vi "Save1DWaveformToFile.vi"(6 "header? (write header:T)":bool=TRUE, 7 "delimiter (Tab)":string="\t", 8 "error in (no error)":errorcluster, 9 "multiple time columns? (single:F)":bool, 10 "waveforms":waveform(dbl)[](array[waveform]), 11 "refnum":refnum<file>) -> (0 "error out":errorcluster, 3 "dup refnum":refnum<file>)   [LabVIEW 2022 SP3]
uses:
  <vilib>/Waveform/WDTOps.llb/WDT Get Waveform Time Array DBL.vi
panel:
  out "spreadsheet string":string
  out "Array":string[](array[string])
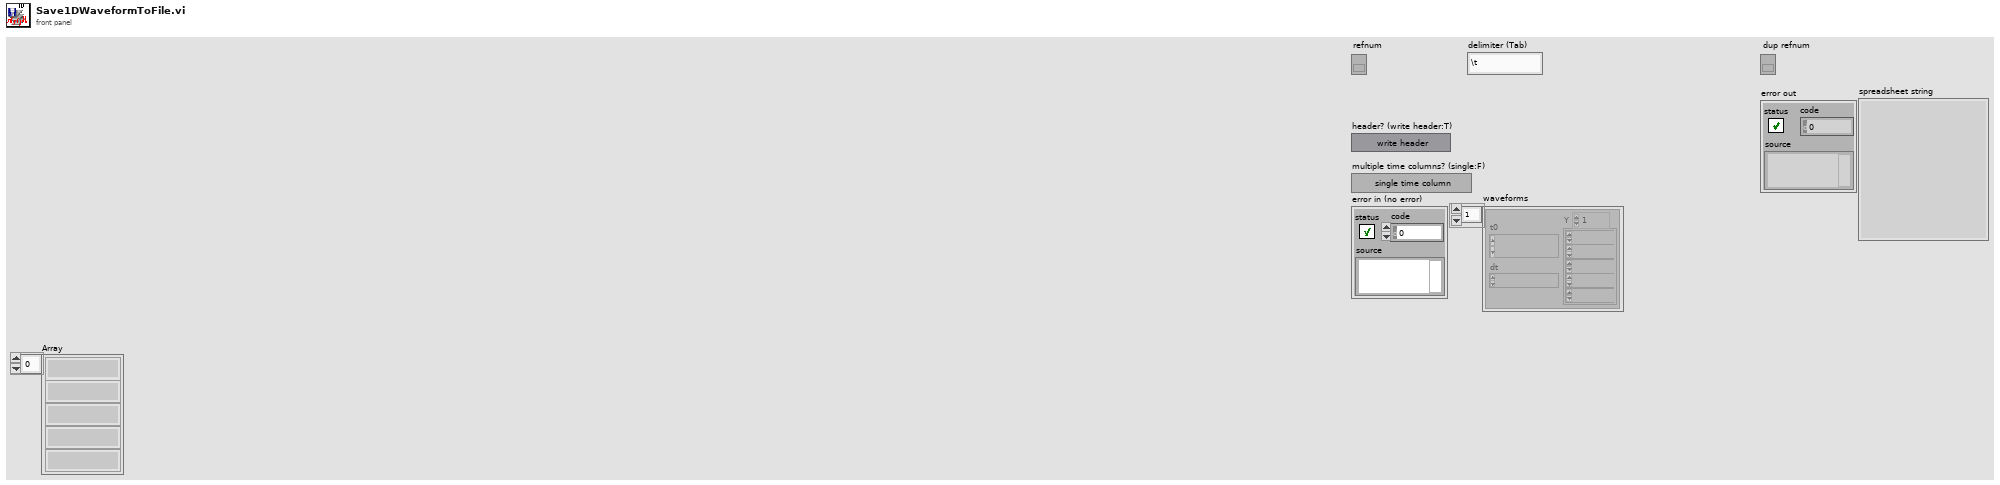
[diagram p1: front panel]
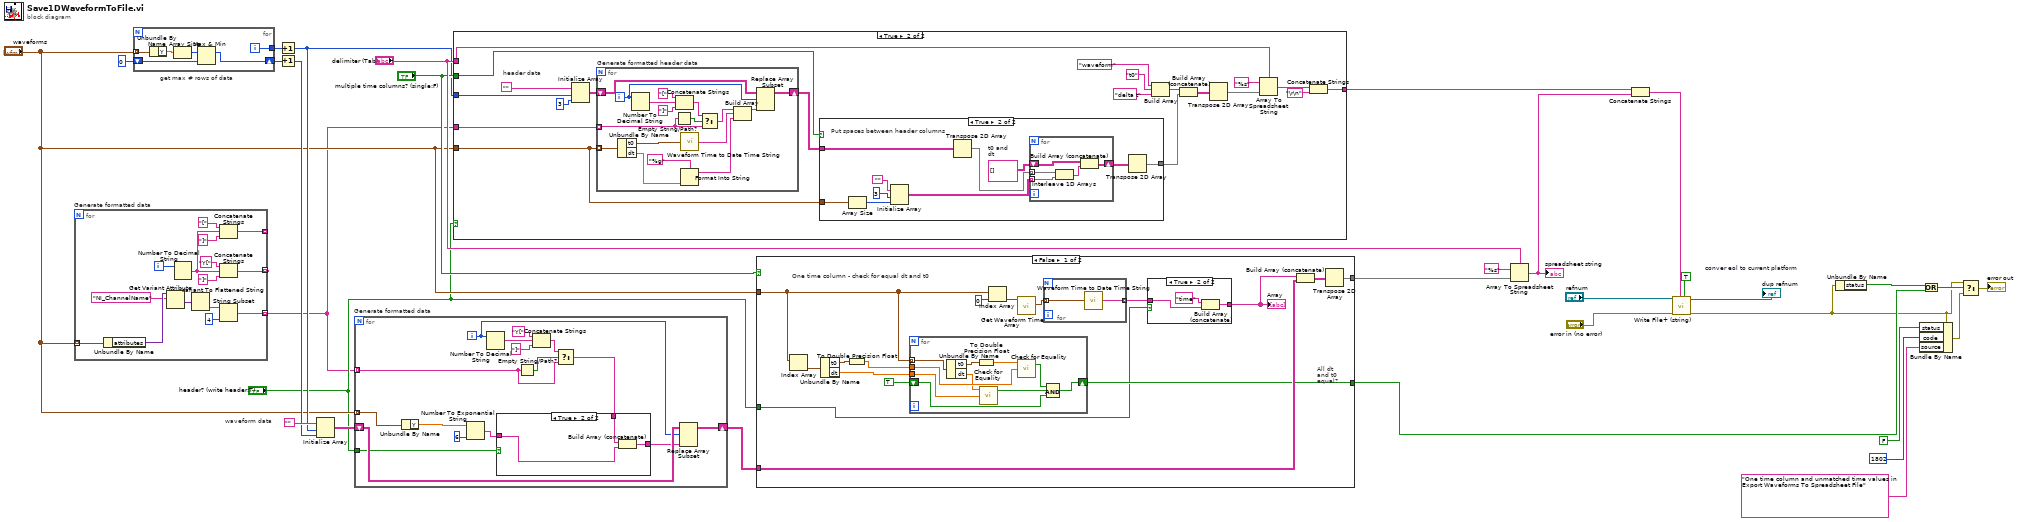
[diagram p0: block diagram]
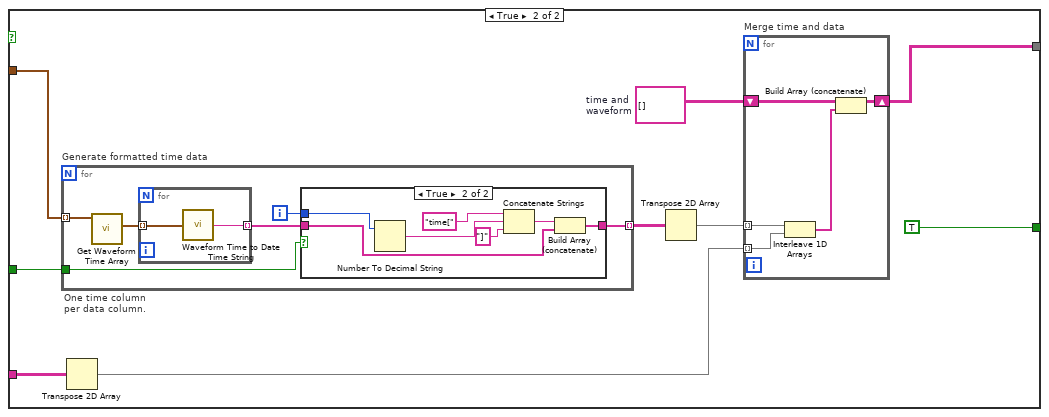
[diagram p3: hidden frame]
diagram:
  w30 = TRUE  # conver eol to current platform
  # "waveform data"
  # "get max # rows of data"
  n1 = for "Generate formatted data" {
    tunnel: "waveforms" -> [w46] mode=indexing
    tunnel: [w37] -> _ mode=indexing
    tunnel: [w36] -> w4 mode=indexing
    tunnel: [w32] -> _ mode=indexing
    i -> [w38]
    n2 = Unbundle By Name(w46) -> ("attributes"=w43:variant)
    n3 = Get Variant Attribute(Variant=w43, name="NI_ChannelName") -> (value=w41:variant)  [unwired: 2 in, 3 out]
    n4 = Number To Decimal String(number=w38) -> (decimal integer string=w33:string)  [unwired: 1 in]
    n5 = Variant To Flattened String(Variant=w41) -> (data string=w44:string)  [unwired: 1 out]
    n6 = String Subset(string=w44, offset (0)=4) -> (substring=w36:string)  [unwired: 1 in]
    n7 = Concatenate Strings("[", w33, "]") -> (w32:string)
    n8 = Concatenate Strings("Y[", w33, "]") -> (w37:string)
  }
  n9 = for {
    tunnel: "waveforms" -> [w52] mode=indexing
    shift-right: [w48] -> w11
    shift-left: 0 -> [w49]
    tunnel: [w47] -> w9
    i -> [w47]
    n10 = Unbundle By Name(w52) -> ("Y"=w51:dbl[])
    n11 = Array Size(array=w51) -> (size(s)=w50:i32)
    n12 = Max & Min(x=w50, y=w49) -> (max(x,y)=w48:i32)  [unwired: 1 out]
  }
  n13 = Increment(x=w9) -> (x+1=w8:i32)
  n14 = Increment(x=w11) -> (x+1=w7:i32)
  n15 = Initialize Array("", w8, w7) -> (w10:string[][])
  n16 = for "Generate formatted data" {
    tunnel: "waveforms" -> [w66] mode=indexing
    tunnel: "header? (write header:T)" -> [w63]
    shift-right: [w64] -> w24
    shift-left: w10 -> [w65]
    tunnel: w4 -> [w53] mode=indexing
    i -> [w55]
    n17 = Unbundle By Name(w66) -> ("Y"=w68:dbl[])
    n18 = Number To Exponential String(number=w68, precision (6)=i16 6) -> (E-format string=w62:string[])  [unwired: 2 in]
    n19 = Number To Decimal String(number=w55) -> (decimal integer string=w60:string)  [unwired: 1 in]
    n20 = Empty String/Path?(string/path=w53) -> (empty?=w57:bool)
    n21 = Concatenate Strings("Y[", w60, "]") -> (w54:string)
    n22 = Select(t=w54, s=w57, f=w53) -> (s? t:f=w56:string)
    n23 = case shown="True" w63 {
      tunnel: w62 -> [w69 w72]
      tunnel: [w69 w71] -> w61
      tunnel: w56 -> [_ w70]
      frame False {
      }
      frame True {
        n24 = Build Array (concatenate)(w70, w72) -> (w71:string[])
      }
    }
    n25 = Replace Array Subset(array=w65, new element=w61, index (row)=w55) -> (w64:string[][])  [unwired: 1 in]
  }
  n26 = case shown="True" "header? (write header:T)" {
    tunnel: "delimiter (Tab)" -> [_ w90]
    tunnel: "waveforms" -> [_ w84]
    tunnel: [_ w85] -> w25
    tunnel: "multiple time columns? (single:F)" -> [_ w82]
    tunnel: w8 -> [_ w75]
    tunnel: w4 -> [_ w73]
    frame False {
    }
    frame True {
      # "header data"
      n27 = Initialize Array("", w75, 3 ("dimension size")) -> (w74:string[][])
      n28 = for "Generate formatted header data" {
        tunnel: w84 -> [w119] mode=indexing
        shift-right: [w114] -> w80
        shift-left: w74 -> [w115]
        tunnel: w73 -> [w109] mode=indexing
        i -> [w113]
        n29 = Unbundle By Name(w119) -> ("t0"=w117:timestamp, "dt"=w123:dbl)
        n30 = Number To Decimal String(number=w113) -> (decimal integer string=w122:string)  [unwired: 1 in]
        n31 = Concatenate Strings("[", w122, "]") -> (w112:string)
        n32 = Empty String/Path?(string/path=w109) -> (empty?=w110:bool)
        n33 = call <vilib>:"Waveform Time to Date Time String.vi"("t0"=w117) -> ("String"=w124:string)
        n34 = Format Into String(format string="%g" ("Format String"), w123) -> (resulting string=w125:string)  [unwired: 2 in, 1 out]
        n35 = Select(t=w112, s=w110, f=w109) -> (s? t:f=w111:string)
        n36 = Build Array(w111, w124, w125) -> (w116:string[])
        n37 = Replace Array Subset(array=w115, new element=w116, index (row)=w113) -> (w114:string[][])  [unwired: 1 in]
      }
      n38 = case shown="True" w82 {
        tunnel: w84 -> [_ w103]
        tunnel: [w93 w98] -> w81
        tunnel: w80 -> [w93 w97]
        frame False {
          # "Leave the header data alone"
        }
        frame True {
          w101 = string[][] []  # t0 and dt
          # "Put spaces between header columns"
          n39 = Array Size(array=w103) -> (size(s)=w94:i32)
          n40 = Initialize Array("", 3 ("Dimension Size"), w94) -> (w100:string[][])
          n41 = Transpose 2D Array(2D array=w97) -> (transposed array=w96:string[][])
          n42 = for {
            shift-right: [w105] -> w99
            shift-left: w101 -> [w106]
            tunnel: w100 -> [w108] mode=indexing
            tunnel: w96 -> [w104] mode=indexing
            n43 = Interleave 1D Arrays(w104, w108) -> (w107:string[])
            n44 = Build Array (concatenate)(w106, w107) -> (w105:string[][])
          }
          n45 = Transpose 2D Array(2D array=w99) -> (transposed array=w98:string[][])
        }
      }
      n46 = Build Array("waveform", "t0", "delta t") -> (w83:string[])
      n47 = Build Array (concatenate)(w83, w81) -> (w78:string[][])
      n48 = Transpose 2D Array(2D array=w78) -> (transposed array=w79:string[][])
      n49 = Array To Spreadsheet String(delimiter (Tab)=w90, array=w79, 3:"%s" ("format string")) -> (spreadsheet string=w87:string)
      n50 = Concatenate Strings(w87, "\r\n") -> (w85:string)
    }
  }
  n51 = case shown="False" "multiple time columns? (single:F)" {
    tunnel: "waveforms" -> [w130 w166]
    tunnel: w24 -> [w137 w164]
    tunnel: [w135 w160] -> w23
    tunnel: [w129 TRUE] -> w14
    tunnel: "header? (write header:T)" -> [w126 w158]
    frame False {
      # "One time column - check for equal dt and t0"
      # "All dt\nand t0\nequal?"
      n52 = Index Array(array=w130) -> (element=w134:waveform(dbl))  [unwired: 1 in]
      n53 = Unbundle By Name(w134) -> ("t0"=w128:timestamp, "dt"=w131:dbl)
      n54 = To Double Precision Float(number=w128) -> (double precision float=w132:dbl)
      n55 = for {
        tunnel: w130 -> [w155] mode=indexing
        shift-right: [w150] -> w129
        shift-left: TRUE -> [w149]
        tunnel: w132 -> [w153]
        tunnel: w131 -> [w151]
        n56 = Unbundle By Name(w155) -> ("t0"=w146:timestamp, "dt"=w152:dbl)
        n57 = To Double Precision Float(number=w146) -> (double precision float=w154:dbl)
        n58 = call <vilib>:"Check for Equality.vi"("n2"=w151, "n1"=w152) -> ("equal?"=w148:bool)  [unwired: 1 in, 1 out]
        n59 = call <vilib>:"Check for Equality.vi"("n2"=w153, "n1"=w154) -> ("equal?"=w147:bool)  [unwired: 1 in, 1 out]
        n60 = Compound Arithmetic op=AND(w147, w148, w149) -> (w150:bool)
      }
      n61 = Index Array(array=w130, index=0 ("Index")) -> (element=w139:waveform(dbl))
      n62 = call-poly <vilib>:"Get Waveform Time Array.vi"("waveform in"=w139) -> ("X array"=w141:timestamp[])  [unwired: 9 in, 1 out]
      n63 = for {
        tunnel: w141 -> [w156] mode=indexing
        tunnel: [w157] -> w138 mode=indexing
        n64 = call <vilib>:"Waveform Time to Date Time String.vi"("t0"=w156) -> ("String"=w157:string)
      }
      n65 = case shown="True" w126 {
        tunnel: w138 -> [w142 w145]
        tunnel: [w142 w144] -> w127
        frame False {
        }
        frame True {
          n66 = Build Array (concatenate)("time", w145) -> (w144:string[])
        }
      }
      "Array" <- w127
      n67 = Build Array (concatenate)(w127, w137) -> (w136:string[][])
      n68 = Transpose 2D Array(2D array=w136) -> (transposed array=w135:string[][])
    }
    frame True {
      w161 = string[][] []  # time and waveform
      # "One time column\nper data column."
      n69 = for "Generate formatted time data" {
        tunnel: [w172] -> w165 mode=indexing
        tunnel: w166 -> [w176] mode=indexing
        tunnel: w158 -> [w174]
        i -> [w175]
        n70 = call-poly <vilib>:"Get Waveform Time Array.vi"("waveform in"=w176) -> ("X array"=w177:timestamp[])  [unwired: 9 in, 1 out]
        n71 = for {
          tunnel: w177 -> [w186] mode=indexing
          tunnel: [w187] -> w173 mode=indexing
          n72 = call <vilib>:"Waveform Time to Date Time String.vi"("t0"=w186) -> ("String"=w187:string)
        }
        n73 = case shown="True" w174 {
          tunnel: w175 -> [_ w182]
          tunnel: w173 -> [w178 w180]
          tunnel: [w178 w179] -> w172
          frame False {
          }
          frame True {
            n74 = Number To Decimal String(number=w182) -> (decimal integer string=w185:string)  [unwired: 1 in]
            n75 = Concatenate Strings("time[", w185, "]") -> (w181:string)
            n76 = Build Array (concatenate)(w181, w180) -> (w179:string[])
          }
        }
      }
      n77 = Transpose 2D Array(2D array=w164) -> (transposed array=w163:string[][])
      n78 = Transpose 2D Array(2D array=w165) -> (transposed array=w162:string[][])
      n79 = for "Merge time and data" {
        tunnel: w163 -> [w170] mode=indexing
        tunnel: w162 -> [w169] mode=indexing
        shift-right: [w168] -> w160
        shift-left: w161 -> [w171]
        n80 = Interleave 1D Arrays(w169, w170) -> (w167:string[])
        n81 = Build Array (concatenate)(w171, w167) -> (w168:string[][])
      }
    }
  }
  n82 = Array To Spreadsheet String(delimiter (Tab)="delimiter (Tab)", array=w23, 3:"%s" ("format (%.3f)")) -> (spreadsheet string=w27:string)
  "spreadsheet string" <- w27
  n83 = Concatenate Strings(w25, w27) -> (w26:string)
  n84 = call <vilib>:"Write File+ (string).vi"("convert eol? (no:F)"=w30, "string"=w26, "error in (no error)"="error in (no error)", "refnum"="refnum") -> ("error out"=w1:errorcluster, "dup refnum"=→"dup refnum":refnum<file>)  [unwired: 3 in, 1 out]
  n85 = Unbundle By Name(w1) -> ("status"=w20:bool)
  n86 = Bundle By Name(cluster=w1, "status"=FALSE, "code"=1802, "source"="One time column and unmatched time values in Export Waveforms To Spreadsheet File") -> (w21:errorcluster)
  n87 = Or(x=w20, y=w14) -> (x .or. y?=w19:bool)
  n88 = Select(t=w1, s=w19, f=w21) -> (s? t:f=→"error out":errorcluster)
